vi "Memory.Pointer.Internal.Dispose.vi"(8 "error in (no error)":errorcluster, 11 "pointer":refnum<class "Memory.Pointer.Internal.lvclass">) -> (0 "error out":errorcluster)   [LabVIEW 2016, in "Memory Manager.lvlib" / "Memory.Pointer.Internal.lvclass"]
doc: "Disposes of the provided <b>pointer</b> and deallocates the associated memory."
uses:
  Memory.Pointer.Internal.lvclass
  C:/Users/Ryan/Documents/Git/Sourcetree/LabVIEW-Memory-Manager/Source/Library/Classes/Pointer/Memory.Pointer.lvclass
  Pointer/Memory.Pointer.lvclass/Memory.Pointer.ctl
  Pointer/Memory.Pointer.lvclass
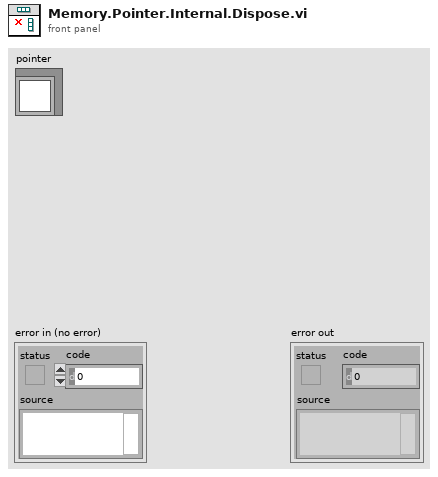
[diagram p1: front panel]
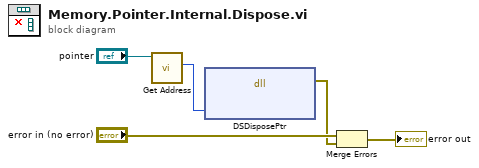
[diagram p0: block diagram]
diagram:
  n1 = call "Get Address.vi"("Pointer in"="pointer") -> ("address"=w5:u64)  [unwired: 8 in, 2 out]
  n2 = dll-call lib="LabVIEW" fn="DSDisposePtr"("pointer"=w5) -> (error out=w2:errorcluster)  [unwired: 5 in, 1 out]
  n3 = Merge Errors("error in (no error)", w2) -> (→"error out":errorcluster)
